vi "Find Target Library.vi"(7 "Library Name":string="Engine.lvlib", 8 "error in (no error)":errorcluster, 10 "Target Name":string="My Computer", 11 "CD Build Tools in":refnum<class "Project Sync Tools.lvclass">) -> (0 "error out":errorcluster, 1 "Found ?":bool, 2 "Library out":refnum<vi>, 3 "CD Build Tools out":refnum<class "Project Sync Tools.lvclass">)   [LabVIEW 2019, in "Project Sync Tools.lvclass"]
uses:
  Project Sync Tools.lvclass
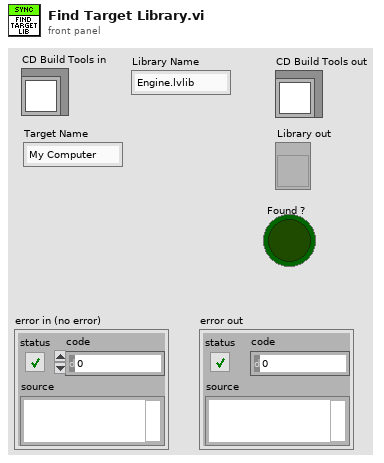
[diagram p1: front panel]
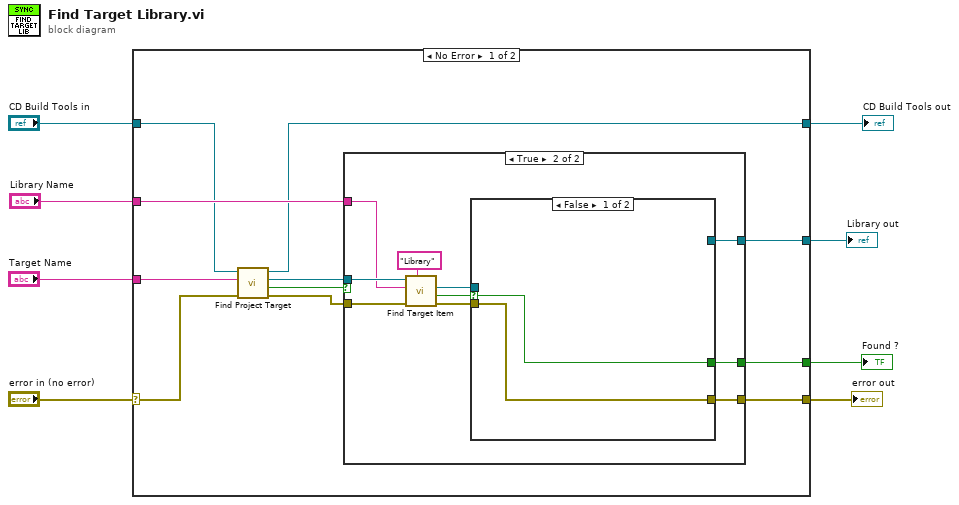
[diagram p0: block diagram]
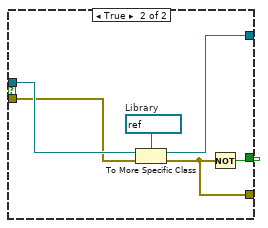
[diagram p3: hidden frame]
diagram:
  n1 = case shown="No Error" "error in (no error)" {
    selector: "error in (no error)" -> [w14 w41]
    tunnel: [w19 w41] -> w8
    tunnel: [w18 _] -> w7
    tunnel: [w13 _] -> w5
    tunnel: "CD Build Tools in" -> [w10 w40]
    tunnel: [w9 w40] -> w3
    tunnel: "Target Name" -> [w12 _]
    tunnel: "Library Name" -> [w11 _]
    frame No Error {
      n2 = call "Find Project Target.vi"("error in (no error)"=w14, "Target Name"=w12, "Project Sync Tools in"=w10) -> ("error out"=w17:errorcluster, "Found ?"=w15:bool, "TargetItem out"=w16:refnum<vi>, "Project Sync Tools out"=w9:refnum<class "Project Sync Tools.lvclass">)  [unwired: 5 in]
      n3 = case shown="True" w15 {
        selector: w15 -> [w20 _]
        tunnel: [w21 w31] -> w19
        tunnel: [_ w30] -> w18
        tunnel: w17 -> [w21 w28]
        tunnel: w16 -> [_ w27]
        tunnel: [w20 w24] -> w13
        tunnel: w11 -> [_ w23]
        frame False {
        }
        frame True {
          n4 = call "Find Target Item.vi"("Type"="Library", "error in (no error)"=w28, "Target Item Name"=w23, "TargetItem in"=w27) -> ("error out"=w26:errorcluster, "Found ?"=w25:bool, "Item out"=w29:refnum<vi>)  [unwired: 4 in, 1 out]
          n5 = case shown="False" w25 {
            selector: w25 -> [w32 _]
            tunnel: [w33 w35] -> w31
            tunnel: [_ w39] -> w30
            tunnel: w29 -> [_ w37]
            tunnel: w26 -> [w33 w34]
            tunnel: [w32 w36] -> w24
            frame False {
            }
            frame True {
              w38 = refnum<vi> refnum  # Library
              n6 = To More Specific Class(target class=w38, reference=w37, error in=w34) -> (specific class reference=w39:refnum<vi>, error out=w35:errorcluster)
              n7 = Not(x=w35) -> (.not. x?=w36:bool)
            }
          }
        }
      }
    }
    frame Error {
    }
  }
  "error out" <- w8
  "Library out" <- w7
  "Found ?" <- w5
  "CD Build Tools out" <- w3
